vi "gen_sine_function.vi"(8 "error in (no error)":errorcluster, 11 "TrajectoryAK101022Resonance in":refnum<class "TrajectoryAK101022Resonance.lvclass">) -> (0 "error out":errorcluster, 1 "z-frequency":dbl[unit], 2 "z-points":dbl[unit][][](array[numeric]), 3 "TrajectoryAK101022Resonance out":refnum<class "TrajectoryAK101022Resonance.lvclass">)   [LabVIEW 2010, in "TrajectoryAK101022Resonance.lvclass"]
uses:
  TrajectoryAK101022Resonance.lvclass
  FPGAWrapper/FPGAWrapperAK101022Resonance/FPGAWrapperAK101022Resonance/FPGAWrapperAK101022Resonance.lvclass
  TrajectoryAK101022Resonance.lvclass/TrajectoryAK101022Resonance.ctl
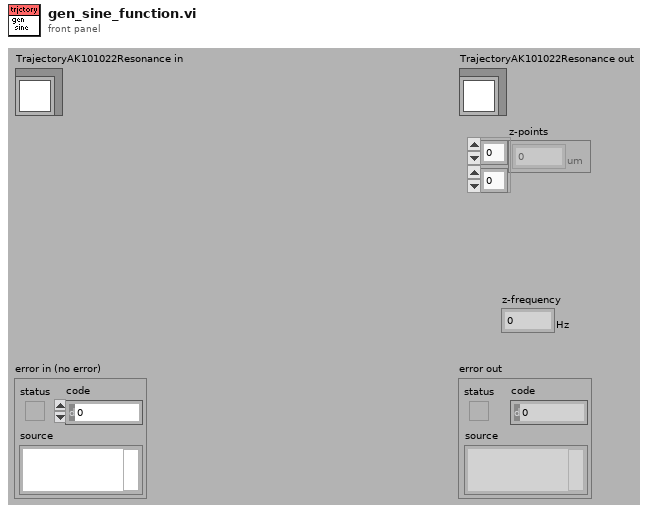
[diagram p1: front panel]
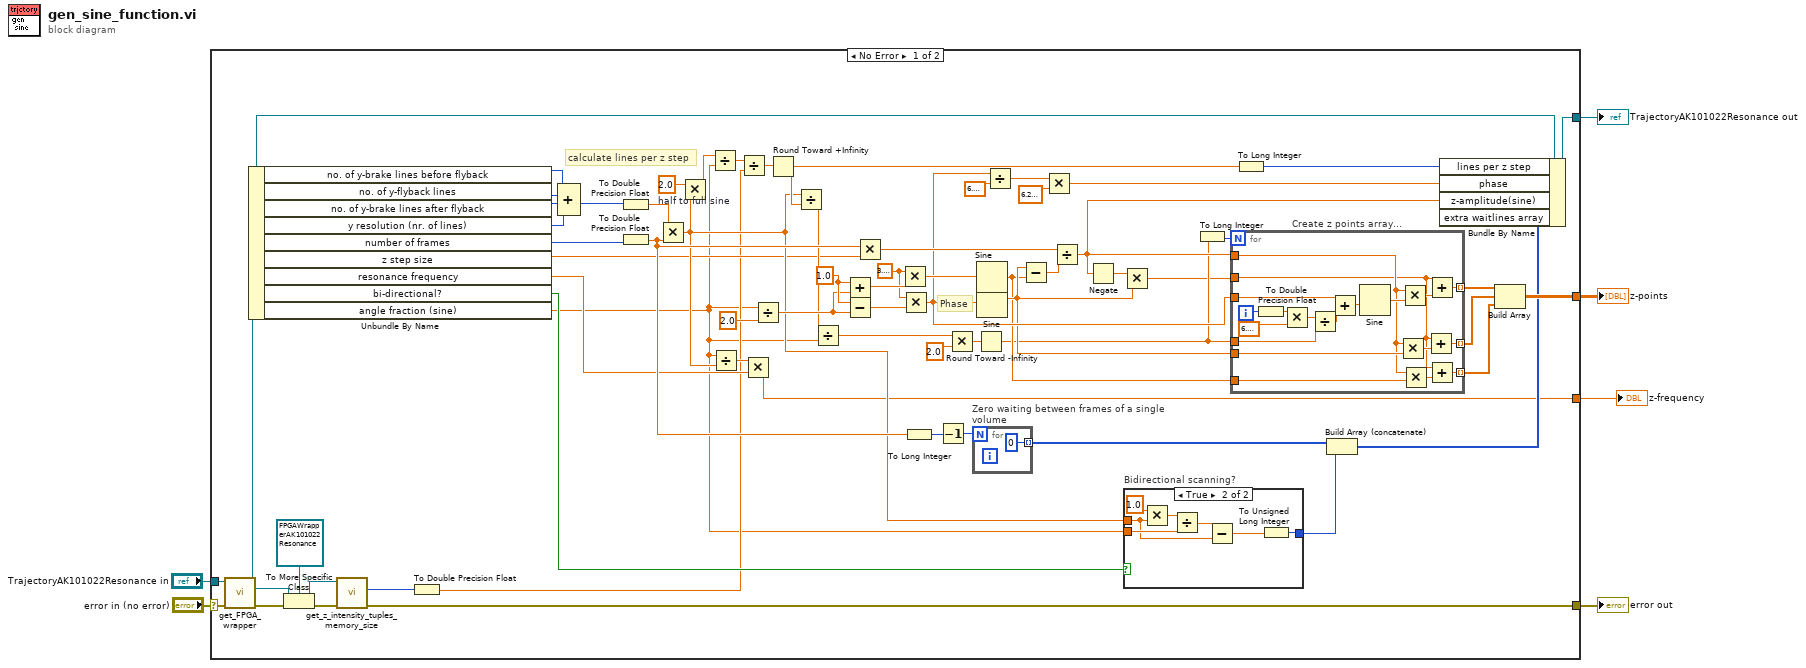
[diagram p0: block diagram]
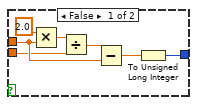
[diagram p2: hidden frame]
diagram:
  n1 = case shown="No Error" "error in (no error)" {
    selector: "error in (no error)" -> [w35 w109]
    tunnel: [w32 w109] -> w5
    tunnel: [w72 w108] -> w4
    tunnel: "TrajectoryAK101022Resonance in" -> [w34 w108]
    tunnel: [w73 _] -> w2
    tunnel: [w8 _] -> w1
    frame No Error {
      w48 = 2.0  # half to full sine
      w70 = 3.141592653589793
      w55 = 1.0
      # "calculate lines per z step"
      # "Phase"
      n2 = call-dynamic "get_FPGA_wrapper.vi"("error in (no error)"=w35, "TrajectoryMG100122GenericFPGA in"=w34) -> ("error out"=w30:errorcluster, "GenericFPGAWrapper.lvclass"=w31:refnum<class "GenericFPGAWrapper.lvclass">, "TrajectoryMG100122GenericFPGA out"=w33:refnum<class "TrajectoryAK101022Resonance.lvclass">)  [unwired: 7 in]
      n3 = Unbundle By Name(w33) -> ("no. of y-brake lines before flyback"=w44:i32, "no. of y-flyback lines"=w43:i32, "no. of y-brake lines after flyback"=w42:i32, "y resolution (nr. of lines)"=w15:i32, "number of frames"=w13:i32, "z step size"=w12:dbl[unit], "resonance frequency"=w16:dbl[unit], "bi-directional?"=w23:bool, "angle fraction (sine)"=w7:dbl)
      n4 = To More Specific Class(target class=refnum<class "FPGAWrapperAK101022Resonance.lvclass"> refnum ("FPGAWrapperAK101022Resonance.lvclass"), reference=w31, error in=w30) -> (specific class reference=w27:refnum<class "FPGAWrapperAK101022Resonance.lvclass">, error out=w29:errorcluster)
      n5 = call "get_z_intensity_tuples_memory_size.vi"("error in (no error)"=w29, "FPGAWrapperAK101022Resonance in"=w27) -> ("error out"=w32:errorcluster, "z/intensity memory size"=w26:i32)  [unwired: 7 in, 1 out]
      n6 = To Double Precision Float(number=w26) -> (double precision float=w11:dbl)
      n7 = Compound Arithmetic op=ADD(w44, w43, w42, w15) -> (w14:i32)
      n8 = To Double Precision Float(number=w14) -> (double precision float=w52:dbl)
      n9 = To Double Precision Float(number=w13) -> (double precision float=w25:dbl)
      n10 = Multiply(x=w52, y=w25) -> (x*y=w18:dbl)
      n11 = Multiply(x=w48, y=w18) -> (x*y=w47:dbl)
      n12 = Divide(x=w47, y=w7) -> (x/y=w49:dbl)
      n13 = Divide(x=w7, y=w18) -> (x/y=w36:dbl)
      n14 = Divide(x=w49, y=w11) -> (x/y=w51:dbl)
      n15 = Multiply(x=w36, y=w16) -> (x*y=w8:dbl[unit])
      n16 = Divide(x=w7, y=2.0) -> (x/y=w54:dbl)
      n17 = Round Toward +Infinity(x=w51) -> (ceil(x): smallest int >= x=w46:dbl)
      n18 = Divide(x=w18, y=w46) -> (x/y=w20:dbl)
      n19 = Divide(x=w20, y=w7) -> (x/y=w64:dbl)
      n20 = Add(x=w55, y=w54) -> (x+y=w71:dbl)
      n21 = Subtract(x=w55, y=w54) -> (x-y=w69:dbl)
      n22 = Multiply(x=w25, y=w12) -> (x*y=w66:dbl[unit])
      n23 = Multiply(x=w70, y=w71) -> (x*y=w68:dbl)
      n24 = Multiply(x=w70, y=w69) -> (x*y=w59:dbl)
      n25 = To Long Integer(number=w25) -> (32bit integer=w22:i32)
      n26 = Decrement(x=w22) -> (x-1=w21:i32)
      n27 = Multiply(x=w64, y=2.0) -> (x*y=w62:dbl)
      n28 = for "Zero waiting between frames of a single volume" {
        N: w21 -> [_]
        tunnel: [u32 0] -> w24 mode=indexing
      }
      n29 = Round Toward -Infinity(1:w62) -> (0:w19:dbl)
      n30 = Sine(x=w68) -> (sin(x)=w40:dbl)
      n31 = Sine(x=w59) -> (sin(x)=w41:dbl)
      n32 = Divide(x=w59, y=6.283185307179586) -> (x/y=w57:dbl)
      n33 = Subtract(x=w41, y=w40) -> (x-y=w67:dbl)
      n34 = Multiply(x=w57, y=dbl[unit] 6.283185307179586) -> (x*y=w56:dbl[unit])
      n35 = Divide(x=w66, y=w67) -> (x/y=w45:dbl[unit])
      n36 = Negate(x=w45) -> (-x=w65:dbl[unit])
      n37 = Multiply(x=w65, y=w41) -> (x*y=w10:dbl[unit])
      n38 = case "Bidirectional scanning?" shown="True" w23 {
        tunnel: w18 -> [w76 w82]
        tunnel: [w74 w87] -> w17
        tunnel: w7 -> [w75 w84]
        frame False {
          n39 = Multiply(x=2.0, y=w76) -> (x*y=w79:dbl)
          n40 = Divide(x=w79, y=w75) -> (x/y=w78:dbl)
          n41 = Subtract(x=w78, y=w76) -> (x-y=w77:dbl)
          n42 = To Unsigned Long Integer(number=w77) -> (unsigned 32bit integer=w74:u32)
        }
        frame True {
          n43 = Multiply(x=1.0, y=w82) -> (x*y=w85:dbl)
          n44 = Divide(x=w85, y=w84) -> (x/y=w83:dbl)
          n45 = Subtract(x=w83, y=w82) -> (x-y=w81:dbl)
          n46 = To Unsigned Long Integer(number=w81) -> (unsigned 32bit integer=w87:u32)
        }
      }
      n47 = To Long Integer(number=w19) -> (32bit integer=w61:i32)
      n48 = for "Create z points array..." {
        N: w61 -> [_]
        tunnel: w19 -> [w106]
        tunnel: w45 -> [w93]
        tunnel: w59 -> [w99]
        tunnel: w10 -> [w92]
        tunnel: [w100] -> w39 mode=indexing
        tunnel: w41 -> [w96]
        tunnel: w40 -> [w90]
        tunnel: [w94] -> w38 mode=indexing
        tunnel: [w89] -> w37 mode=indexing
        i -> [w98]
        n49 = To Double Precision Float(number=w98) -> (double precision float=w97:dbl)
        n50 = Multiply(x=w97, y=6.283185307179586) -> (x*y=w107:dbl)
        n51 = Divide(x=w107, y=w106) -> (x/y=w102:dbl)
        n52 = Add(x=w99, y=w102) -> (x+y=w104:dbl)
        n53 = Sine(x=w104) -> (sin(x)=w103:dbl)
        n54 = Multiply(x=w93, y=w96) -> (x*y=w95:dbl[unit])
        n55 = Multiply(x=w93, y=w103) -> (x*y=w101:dbl[unit])
        n56 = Multiply(x=w93, y=w90) -> (x*y=w91:dbl[unit])
        n57 = Add(x=w92, y=w95) -> (x+y=w94:dbl[unit])
        n58 = Add(x=w92, y=w101) -> (x+y=w100:dbl[unit])
        n59 = Add(x=w92, y=w91) -> (x+y=w89:dbl[unit])
      }
      n60 = To Long Integer(number=w46) -> (32bit integer=w50:i32)
      n61 = Build Array (concatenate)(w24, w17) -> (w9:u32[])
      n62 = Bundle By Name(cluster=w33, "lines per z step"=w50, "phase"=w56, "z-amplitude(sine)"=w45, "extra waitlines array"=w9) -> (w72:refnum<class "TrajectoryAK101022Resonance.lvclass">)
      n63 = Build Array(w39, w38, w37) -> (w73:dbl[unit][][])
    }
    frame Error {
    }
  }
  "error out" <- w5
  "TrajectoryAK101022Resonance out" <- w4
  "z-points" <- w2
  "z-frequency" <- w1
